vi "true=disable.vi"(3 "Flag":bool) -> (1 "Disabled":T1(ring))   [LabVIEW 2014, in "Data Manipulation.lvlib"]
uses:
  Data Manipulation.lvlib
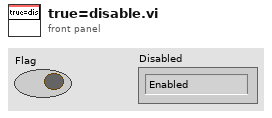
[diagram p1: front panel]
types:
  T1 = enum8{"Enabled", "Disabled", "Disabled and Grayed Out"}
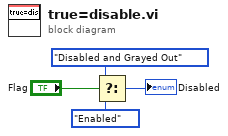
[diagram p0: block diagram]
diagram:
  n1 = Select(t=T1."Disabled and Grayed Out" ("Disabled"), s="Flag", f=T1."Enabled" ("Disabled")) -> (s? t:f=→"Disabled":T1)
